vi "Configure Instrument.vi"(8 "error in (no error)":errorcluster, 11 "Instrument in":refnum<class "Instrument.lvclass">) -> (0 "error out":errorcluster, 3 "Instrument out":refnum<class "Instrument.lvclass">)   [LabVIEW 2016, in "Instrument.lvclass"]
uses:
  Instrument.lvclass
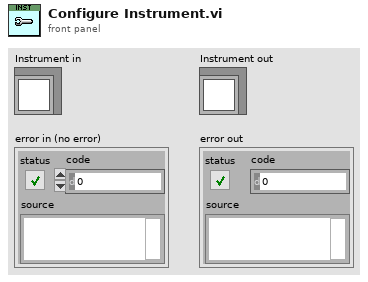
[diagram p1: front panel]
types:
  T1 = typedef "Instrument.lvclass/Configuration--Cluster.ctl" = cluster{"Hardware":T2, "SMO":T3, "DSC":T5}
  T2 = typedef "Instrument.lvclass/HW Configuration--Cluster.ctl" = cluster{"Address":string, "Type":string, "COM Type":string}
  T3 = typedef "Instrument.lvclass/SMO Configuration--Cluster.ctl" = cluster{"Address":string, "Port":u16, "RC Type":T4}
  T4 = typedef "Instrument.lvclass/SMO RC Type--enum.ctl" = enum16{"RC", "STM", "ZMQ"}
  T5 = typedef "Instrument.lvclass/DSC Configuration--Cluster.ctl" = cluster{"Process Name":string}
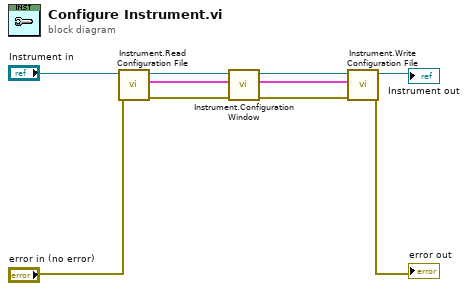
[diagram p0: block diagram]
diagram:
  n1 = call "Instrument.Read Configuration File.vi"("error in (no error)"="error in (no error)", "Instrument in"="Instrument in") -> ("error out"=w4:errorcluster, "Configuration"=w2:T1, "Instrument out"=w3:refnum<class "Instrument.lvclass">)  [unwired: 7 in]
  n2 = call "Instrument.Configuration Window.vi"("error in (no error)"=w4, "Instrument Configuration"=w2, "Instrument in"=w3) -> ("error out"=w6:errorcluster, "output cluster"=w1:T1, "Instrument out"=w5:refnum<class "Instrument.lvclass">)  [unwired: 6 in]
  n3 = call "Instrument.Write Configuration File.vi"("error in (no error)"=w6, "Instrument Configuration"=w1, "Instrument in"=w5) -> ("error out"=→"error out":errorcluster, "Instrument out"=→"Instrument out":refnum<class "Instrument.lvclass">)  [unwired: 7 in]
